vi "mw.vi"(10 "Numeric":dbl, 11 "Frame":i32) -> (1 "output cluster":cluster{"Frame":dbl, "number":dbl})   [LabVIEW 2014]
panel:
  in  "Cluster":cluster{"Frame":dbl, "number":dbl}
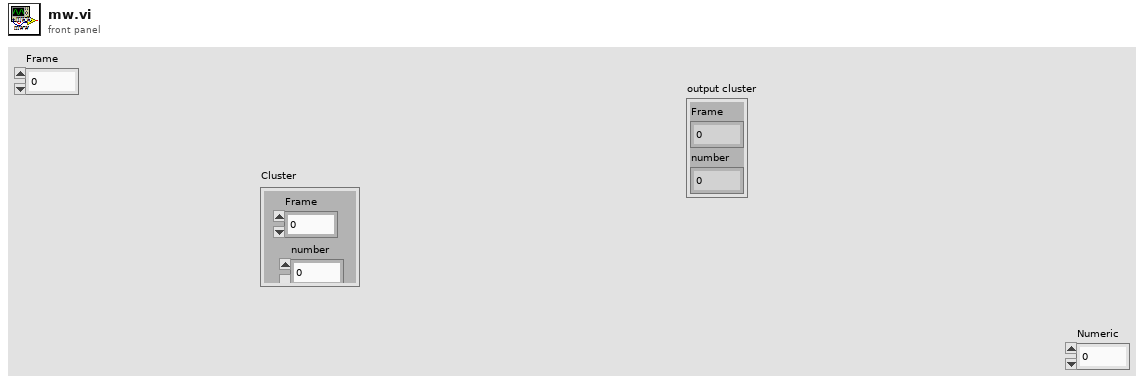
[diagram p1: front panel]
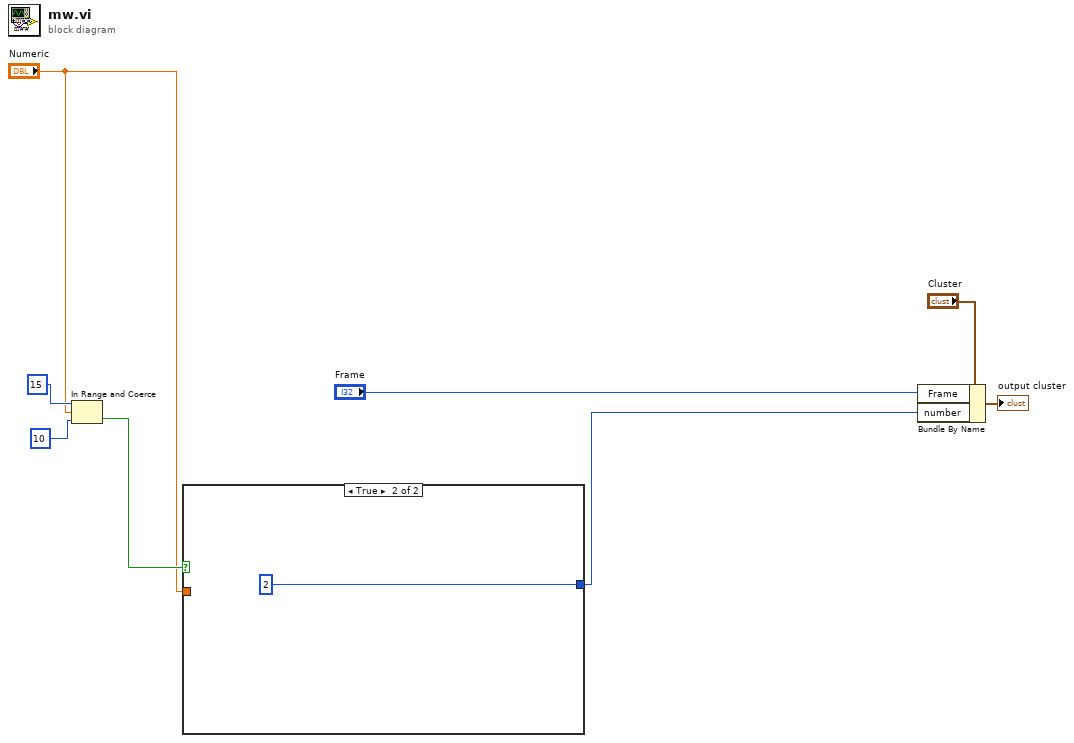
[diagram p0: block diagram]
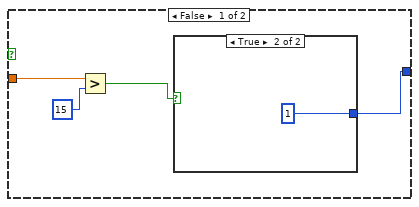
[diagram p2: hidden frame]
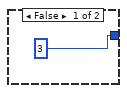
[diagram p3: hidden frame]
diagram:
  n1 = In Range and Coerce(upper limit=15, x="Numeric", lower limit=10) -> (In Range?=w6:bool)  [unwired: 1 out]
  n2 = case shown="True" w6 {
    tunnel: [w9 2] -> w3
    tunnel: "Numeric" -> [w12 _]
    frame False {
      n3 = Greater?(x=w12, y=15) -> (0:w10:bool)
      n4 = case shown="True" w10 {
        tunnel: [3 1] -> w9
        frame False {
        }
        frame True {
        }
      }
    }
    frame True {
    }
  }
  n5 = Bundle By Name(cluster="Cluster", "Frame"="Frame", "number"=w3) -> (→"output cluster":cluster{"Frame":dbl, "number":dbl})
